vi "Read Tags.vi"(8 "error in (no error)":errorcluster, 11 "Tree_LVOOP__lava_lib_tree_class in":refnum<class "Tree Class.lvclass">) -> (0 "error out":errorcluster, 2 "Tags":refnum<class "Tree Tag Class.lvclass">[](array[class]), 3 "Tree_LVOOP__lava_lib_tree_class out":refnum<class "Tree Class.lvclass">)   [LabVIEW 2012, in "Tree Tools.lvlib" / "Tree Class.lvclass"]
uses:
  Tree Class.lvclass
  Tree Tag Class/Tree Tag Class.lvclass
  Tree Class.lvclass/Tree Class.ctl
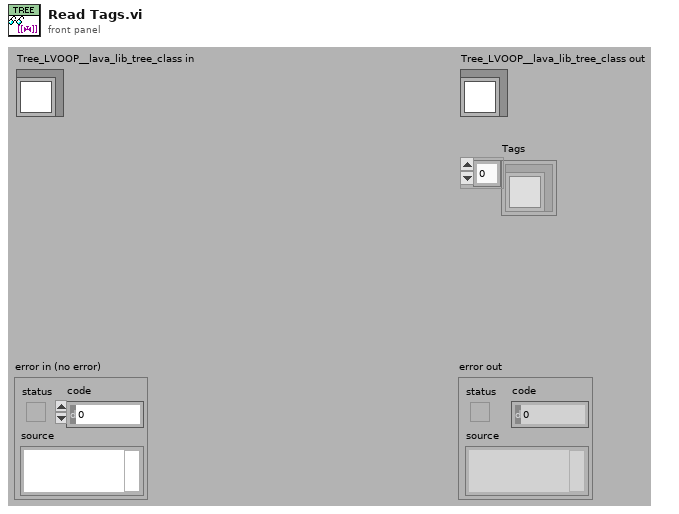
[diagram p1: front panel]
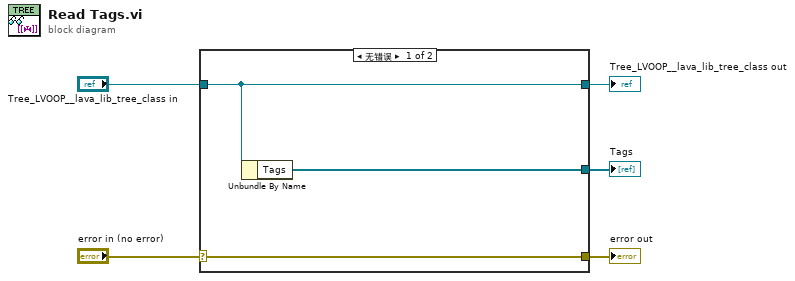
[diagram p0: block diagram]
diagram:
  n1 = case shown="无错误" "error in (no error)" {
    selector: "error in (no error)" -> [w8 w9]
    tunnel: [w8 w9] -> w4
    tunnel: [w7 w10] -> w2
    tunnel: "Tree_LVOOP__lava_lib_tree_class in" -> [w7 w10]
    tunnel: [w6 _] -> w1
    frame No Error {
      n2 = Unbundle By Name(w7) -> ("Tags"=w6:refnum<class "Tree Tag Class.lvclass">[])
    }
    frame Error {
    }
  }
  "error out" <- w4
  "Tree_LVOOP__lava_lib_tree_class out" <- w2
  "Tags" <- w1
